vi "Check in Range.vi"(8 "number of col":i32, 9 "number of rows":i32, 10 "col":i32, 11 "row":i32) -> (3 "in range":bool)   [LabVIEW 2023]
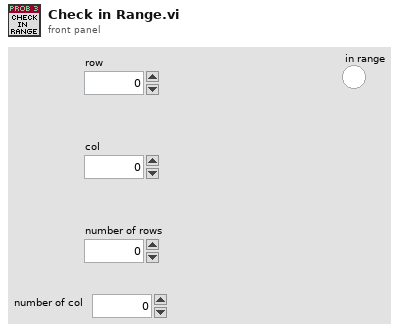
[diagram p1: front panel]
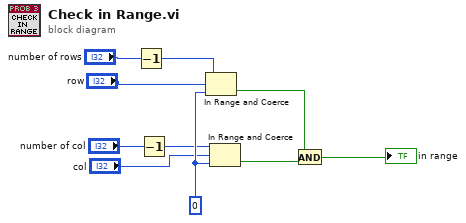
[diagram p0: block diagram]
diagram:
  w6 = 0 ("lower limit")
  n1 = Decrement(x="number of rows") -> (x-1=w7:i32)
  n2 = Decrement(x="number of col") -> (x-1=w5:i32)
  n3 = In Range and Coerce(upper limit=w7, x="row", lower limit=w6) -> (In Range?=w2:bool)  [unwired: 1 out]
  n4 = In Range and Coerce(upper limit=w5, x="col", lower limit=w6) -> (In Range?=w3:bool)  [unwired: 1 out]
  n5 = And(x=w2, y=w3) -> (x .and. y?=→"in range":bool)
